vi "To LabVIEW.vi"(4 "AlbumMap in":refnum<class "VehicleMap.lvclass">, 7 "ExpectedType":refnum<class>, 8 "error in (no error)":errorcluster, 10 "DbRow":variant) -> (0 "error out":errorcluster, 2 "Value":refnum<class>)   [LabVIEW 2020, in "VehicleMap.lvclass"]
uses:
  VehicleMap.lvclass
  C:/Program Files/National Instruments/LabVIEW 2020/vi.lib/Viviota/shared/ORM.lvlibp/ORM/TypeMap/TypeMap.lvclass
  Vehicle/Vehicle.lvclass
  Vehicle/Vehicle.lvclass/Vehicle.ctl
  Vehicle/Write Make.vi
  Vehicle/Write Model.vi
  Vehicle/Write Year.vi
  Vehicle/Write VehicleID.vi
  <vilib>/Viviota/shared/ORM.lvlibp/ORM/TypeMap/Read Autokey.vi
panel:
  out "found":bool
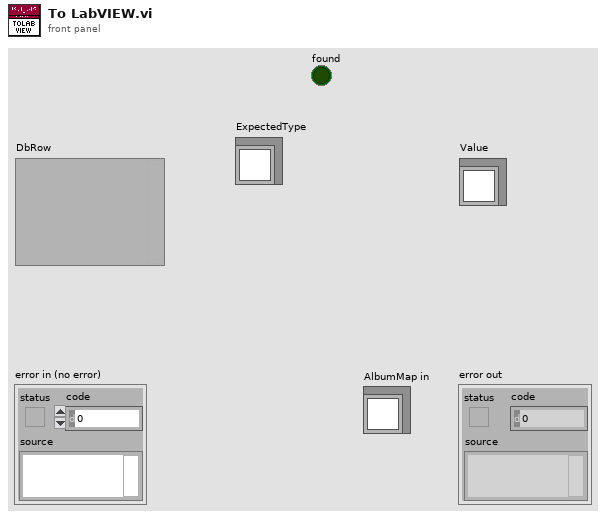
[diagram p1: front panel]
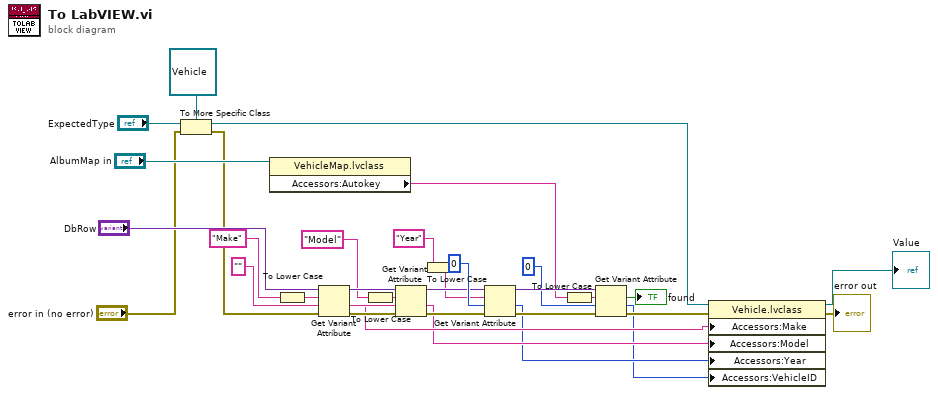
[diagram p0: block diagram]
diagram:
  w22 = "" ("Title")
  n1 = To More Specific Class(target class=refnum<class "Vehicle.lvclass"> refnum ("Vehicle.lvclass"), reference="ExpectedType", error in="error in (no error)") -> (specific class reference=w10:refnum<class "Vehicle.lvclass">, error out=w8:errorcluster)
  n2 = property class="VehicleMap.lvclass"(reference="AlbumMap in") -> ("Accessors:Autokey"=w16:string)  [unwired: 1 in, 2 out]
  n3 = To Lower Case(string="Make" ("Title")) -> (all lower case string=w1:string)
  n4 = Get Variant Attribute(Variant="DbRow", name=w1, default value (empty Variant)=w22, error in=w8) -> (duplicate Variant=w26:variant, value=w21:string, error out=w24:errorcluster)  [unwired: 1 out]
  n5 = To Lower Case(string="Model" ("Title")) -> (all lower case string=w2:string)
  n6 = Get Variant Attribute(Variant=w26, name=w2, default value (empty Variant)=w22, error in=w24) -> (duplicate Variant=w25:variant, value=w20:string, error out=w23:errorcluster)  [unwired: 1 out]
  n7 = To Lower Case(string="Year" ("Title")) -> (all lower case string=w4:string)
  n8 = Get Variant Attribute(Variant=w25, name=w4, default value (empty Variant)=0 ("Primary Key"), error in=w23) -> (duplicate Variant=w17:variant, value=w19:i32, error out=w32:errorcluster)  [unwired: 1 out]
  n9 = To Lower Case(string=w16) -> (all lower case string=w3:string)
  n10 = Get Variant Attribute(Variant=w17, name=w3, default value (empty Variant)=0, error in=w32) -> (found=→"found":bool, value=w15:i32, error out=w18:errorcluster)  [unwired: 1 out]
  n11 = property class="Vehicle.lvclass"(reference=w10, error in=w18, "Accessors:Make"=w21, "Accessors:Model"=w20, "Accessors:Year"=w19, "Accessors:VehicleID"=w15) -> (reference out=→"Value":refnum<class "Vehicle.lvclass">, error out=→"error out":errorcluster)
